vi "Active Write.vi"(4 "error in (no error)":errorcluster, 5 "Value":bool[](array[boolean]), 6 "Container State":T2, 7 "Display State In":T1) -> (0 "error out":errorcluster, 3 "Display State Out":T1)   [LabVIEW 2015, in "Tau.xctl"]
uses:
  Tau.xctl
  <vilib>/_xctls/Container State.ctl
  State.ctl
  <vilib>/_xctls/XControlSupport.lvlib
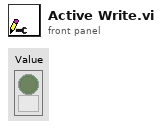
[diagram p1: front panel]
types:
  T1 = typedef "Tau.xctl/State.ctl" = cluster{"Data Array":sgl[][], "Time Array":timestamp[], "History":u16, "Variable":bool[], "Plot Details":cluster{"Name":string, "Line Width":u8, "Line Style":u8, "Color":u32}[]}
  T2 = typedef "XControlSupport.lvlib/Container State.ctl" = cluster{"Indicator?":bool, "Run Mode?":bool, " Refnum":refnum<vi>}
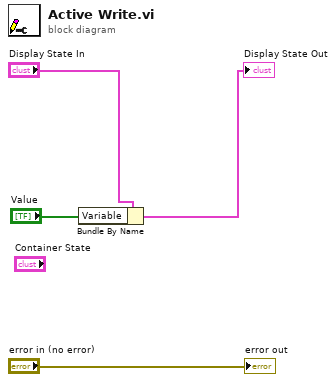
[diagram p0: block diagram]
diagram:
  n1 = Bundle By Name(cluster="Display State In", "Variable"="Value") -> (→"Display State Out":T1)
  "error out" <- "error in (no error)"
